vi "IviLxiSyncConfigureTriggerSource.vi"(7 "Detection (Rise)":i32(ring) items=["Rise", "Fall", "High", "Low"], 8 "error in (no error)":errorcluster {"code" format="%.0x"}, 9 "Delay":dbl caption="Delay (sec)", 10 "SourceName":string="TriggerSource_LXI0" caption="SourceName (TriggerSource_LXI0)", 11 "instrument handle":refnum<k15>) -> (0 "error out":errorcluster {"code" format="%.0x"}, 3 "instrument handle out":refnum<k15>)   [LabVIEW 2009, in "Keysight XSAn.lvlib"]
doc: "This VI configures the most commonly configured properties of the trigger source sub-system.\n\nSupported Models: N9000A, N9000B, N9010A, N9010B, N9020A, N9020B, N9030A, N9030B, N9038A, SPN9003A, SPN9026A"
uses:
  <instrlib>/Keysight XSAn/Keysight XSAn.lvlib
  AgXSAn.dll
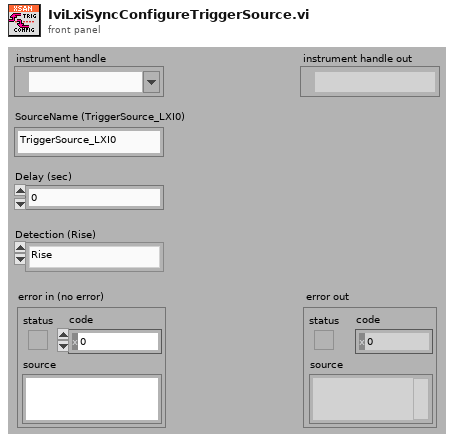
[diagram p1: front panel]
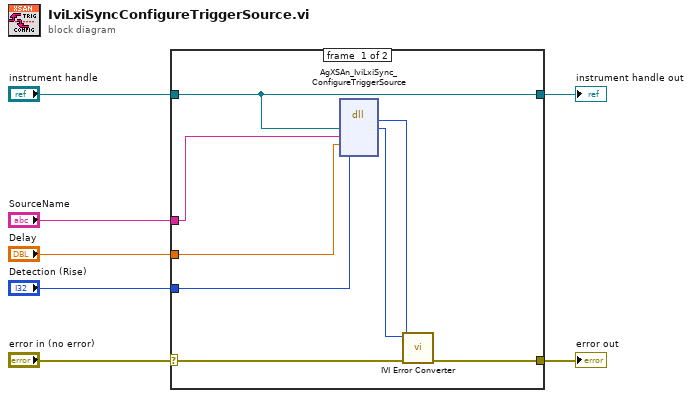
[diagram p0: block diagram]
diagram:
  n1 = case shown="No Error" "error in (no error)" {
    selector: "error in (no error)" -> [w13 w17]
    tunnel: [w12 w17] -> w7
    tunnel: "instrument handle" -> [w8 w16]
    tunnel: "SourceName" -> [w11 _]
    tunnel: "Delay" -> [w10 _]
    tunnel: "Detection (Rise)" -> [w9 _]
    tunnel: [w8 w16] -> w1
    frame #0 {
      n2 = dll-call lib="AgXSAn**.dll" fn="AgXSAn_IviLxiSync_ConfigureTriggerSource"("Vi"=w8, "SourceName"=w11, "Delay"=w10, "Detection"=w9) -> (w14:i32, "Vi"=w15:u32)  [unwired: 6 in, 2 out]
      n3 = call <instrlib>:"IVI Error Converter.vi"("error in (no error)"=w13, "IVI error code (0)"=w14, "instrument handle"=w15) -> ("error out"=w12:errorcluster)  [unwired: 7 in, 1 out]
    }
    frame #1 {
    }
  }
  "error out" <- w7
  "instrument handle out" <- w1
